vi "NI Read Version and Revision Fields from XLSX File.vi"(8 "error in":errorcluster, 11 "XLSX File":path) -> (0 "error out":errorcluster)   [LabVIEW 2018]
doc: "Reads all sheets from the specified <b>XLSX File</b>. This VI does <b>not</b> require Microsoft Excel to be installed.\n\nEach sheet is returned as a 2D Array of Strings. You will need to perform additional conversion if you require data in numeric format.\n\nTime data (date and/or time) is returned as a number of days elapsed since January 1, 1900. Hour/minute/second information will be returned as a fraction of a day (24 hours)."
uses:
  <vilib>/zip/NI_Unzip.lvlib
panel:
  out "Revision String":string
  out "Version String":string
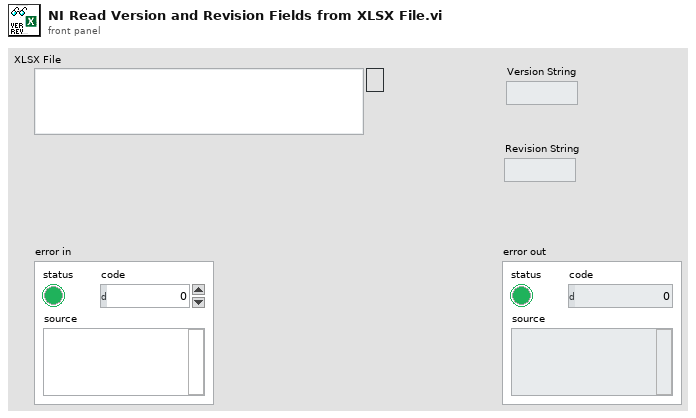
[diagram p1: front panel]
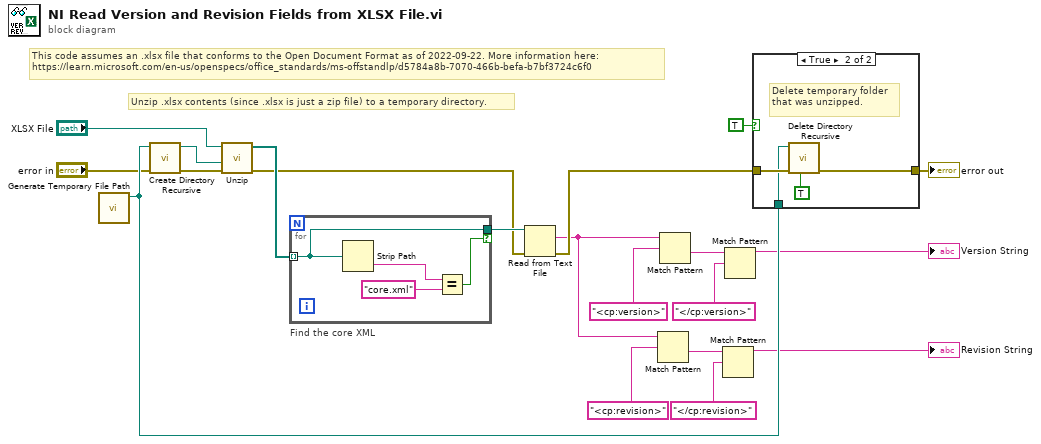
[diagram p0: block diagram]
diagram:
  # "Unzip .xlsx contents (since .xlsx is just a zip file) to a temporary directory."
  # "This code assumes an .xlsx file that conforms to the Open Document Format as of 2022-09-22. More information here:\nhttps://learn.microsoft.com/en-us/openspecs/office_standards/ms-offstandlp/d5784a8b-7070-466b-befa-b7bf3724c6f0"
  n1 = call <vilib>:"Generate Temporary File Path.vi"() -> ("Unique Temporary File Path"=w15:path)  [unwired: 10 in, 1 out]
  n2 = call <vilib>:"Create Directory Recursive.vi"("error in (no error)"="error in", "directory"=w15) -> ("error out"=w20:errorcluster, "directory copy"=w16:path)  [unwired: 3 in, 1 out]
  n3 = call <vilib>:"Unzip.vi"("error in (no error)"=w20, "Target directory (same as Zip file if empty)"=w16, "Zip file"="XLSX File") -> ("error out"=w11:errorcluster, "Unzipped files"=w17:path[])  [unwired: 6 in, 1 out]
  n4 = for "Find the core XML" {
    tunnel: w17 -> [w22] mode=indexing
    tunnel: [w22] -> w12 if=w23
    n5 = Strip Path(path=w22) -> (name=w21:string)  [unwired: 1 out]
    n6 = Equal?(x=w21, y="core.xml") -> (x = y?=w23:bool)
  }
  n7 = Read from Text File(file (use dialog)=w12, error in=w11) -> (text=w2:string, error out=w10:errorcluster)  [unwired: 2 in, 2 out]
  n8 = Match Pattern(string=w2, regular expression="<cp:revision>") -> (after substring=w3:string)  [unwired: 1 in, 3 out]
  n9 = Match Pattern(string=w2, regular expression="<cp:version>") -> (after substring=w9:string)  [unwired: 1 in, 3 out]
  n10 = Match Pattern(string=w3, regular expression="</cp:revision>") -> (before substring=→"Revision String":string)  [unwired: 1 in, 3 out]
  n11 = Match Pattern(string=w9, regular expression="</cp:version>") -> (before substring=→"Version String":string)  [unwired: 1 in, 3 out]
  n12 = case shown="True" TRUE {
    tunnel: w10 -> [w25 w29]
    tunnel: [w25 w28] -> w19
    tunnel: w15 -> [_ w27]
    frame False {
      # "Keep temporary unzip files for debugging"
    }
    frame True {
      # "Delete temporary folder that was unzipped."
      n13 = call <vilib>:"Delete Directory Recursive.vi"("keep deleting on error? (F)"=TRUE, "error in (no error)"=w29, "Folder to Delete"=w27) -> ("error out"=w28:errorcluster)  [unwired: 7 in, 1 out]
    }
  }
  "error out" <- w19
